vi "Initialize.vi"(8 "error in (no error)":errorcluster, 9 "Marca":string, 10 "Puerto Com":refnum<visa-resource-name>, 11 "object in":refnum<class "NXP.lvclass">) -> (0 "error out":errorcluster, 3 "object out":refnum<class "NXP.lvclass">)   [LabVIEW 2020, in "NXP.lvclass"]
doc: "Se inicializa la comunicacion con el nxp de manera serial"
uses:
  NXP.lvclass
  NXP.lvclass/NXP.ctl
  <vilib>/Instr/_visa.llb/VISA Configure Serial Port (Instr).vi
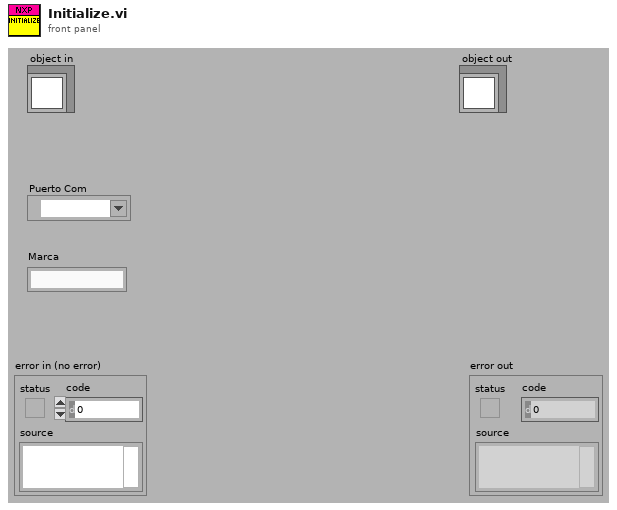
[diagram p1: front panel]
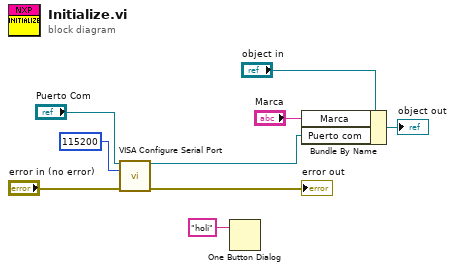
[diagram p0: block diagram]
diagram:
  n1 = call-poly "VISA Configure Serial Port"("VISA resource name"="Puerto Com", "baud rate (9600)"=u32 115200, "error in (no error)"="error in (no error)") -> ("VISA resource name out"=w7:refnum<visa-resource-name>, "error out"=→"error out":errorcluster)  [unwired: 11 in]
  n2 = One Button Dialog(message="holi") -> ()  [unwired: 1 in, 1 out]
  n3 = Bundle By Name(cluster="object in", "Marca"="Marca", "Puerto com"=w7) -> (→"object out":refnum<class "NXP.lvclass">)
